vi "Atto DRY Interface get Vti Heater Power.vi"(8 "error in (no error)":errorcluster, 11 "VTIHeaterPowerW":sgl) -> (0 "error out":errorcluster, 2 "function return":i32, 3 "VTIHeaterPowerW out":sgl)   [LabVIEW 2016, in "attoDRYLib.lvlib"]
doc: "int32_t __cdecl AttoDRY_Interface_getVtiHeaterPower(float *VTIHeaterPowerW);"
uses:
  <userlib>/attoDRYLib/attoDRYLib.lvlib
  <userlib>/attoDRYLib/attoDRYLib.dll
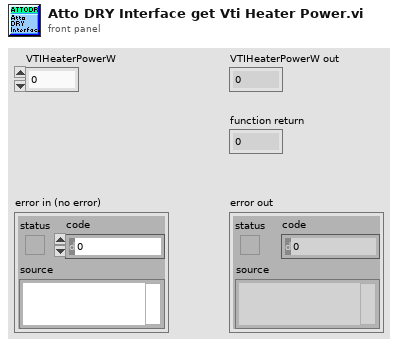
[diagram p1: front panel]
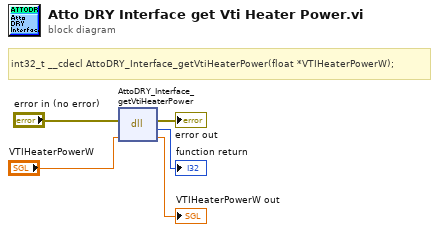
[diagram p0: block diagram]
diagram:
  # "int32_t __cdecl AttoDRY_Interface_getVtiHeaterPower(float *VTIHeaterPowerW);"
  n1 = dll-call lib="C:/Program Files (x86)/National Instruments/LabVIEW 2016/user.lib/attoDRYLib/attoDRYLib.*" fn="AttoDRY_Interface_getVtiHeaterPower"(error in="error in (no error)", "VTIHeaterPowerW"="VTIHeaterPowerW") -> (error out=→"error out":errorcluster, →"function return":i32, "VTIHeaterPowerW"=→"VTIHeaterPowerW out":sgl)  [unwired: 2 in, 1 out]
